vi "niFpga wdp fft DIT 16spc.vi"(0 "real data in":fxp<+/-,8,1>[](array[numeric])=[0.0, 0.0, 0.0, 0.0, 0.0, 0.0, 0.0, 0.0, 0.0, 0.0, 0.0, 0.0, 0.0, 0.0, 0.0, 0.0], 5 "imaginary data in":fxp<+/-,8,1>[](array[numeric])=[0.0, 0.0, 0.0, 0.0, 0.0, 0.0, 0.0, 0.0, 0.0, 0.0, 0.0, 0.0, 0.0, 0.0, 0.0, 0.0], 9 "input frame start":bool, 12 "enable":bool) -> (3 "data indices":u16[](array[numeric]), 4 "real data out":fxp<+,8,1>[](array[numeric]), 6 "imaginary data out":fxp<+,8,1>[](array[numeric]), 10 "output valid":bool, 14 "ready for frame":bool, 15 "output frame start":bool)   [LabVIEW 2017]
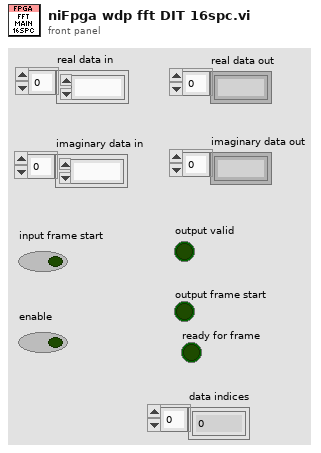
[diagram p1: front panel]
types:
  T1 = cluster{"internal input type":fxp<+/-,8,1>, "internal input type":fxp<+/-,8,1>}
  T2 = cluster{"twiddle factor type":fxp<+/-,16,2>, "twiddle factor type":fxp<+/-,16,2>}[]
  T3 = cluster{"x-y":fxp<+/-,19,12>, "x-y":fxp<+/-,19,12>}
  T4 = cluster{"x+y":fxp<+/-,19,12>, "x+y":fxp<+/-,19,12>}
  T5 = cluster{"x-y":fxp<+/-,19,12>, "x-y":fxp<+/-,19,12>}[]
  T6 = cluster{"x+y":fxp<+/-,19,12>, "x+y":fxp<+/-,19,12>}[]
  T7 = cluster{"data re":fxp<+/-,8,1>, "data im":fxp<+/-,8,1>}[]
  T8 = cluster{"x-y":fxp<+/-,20,13>, "x-y":fxp<+/-,20,13>}[]
  T9 = cluster{"x-y":fxp<+/-,20,13>, "x-y":fxp<+/-,20,13>}
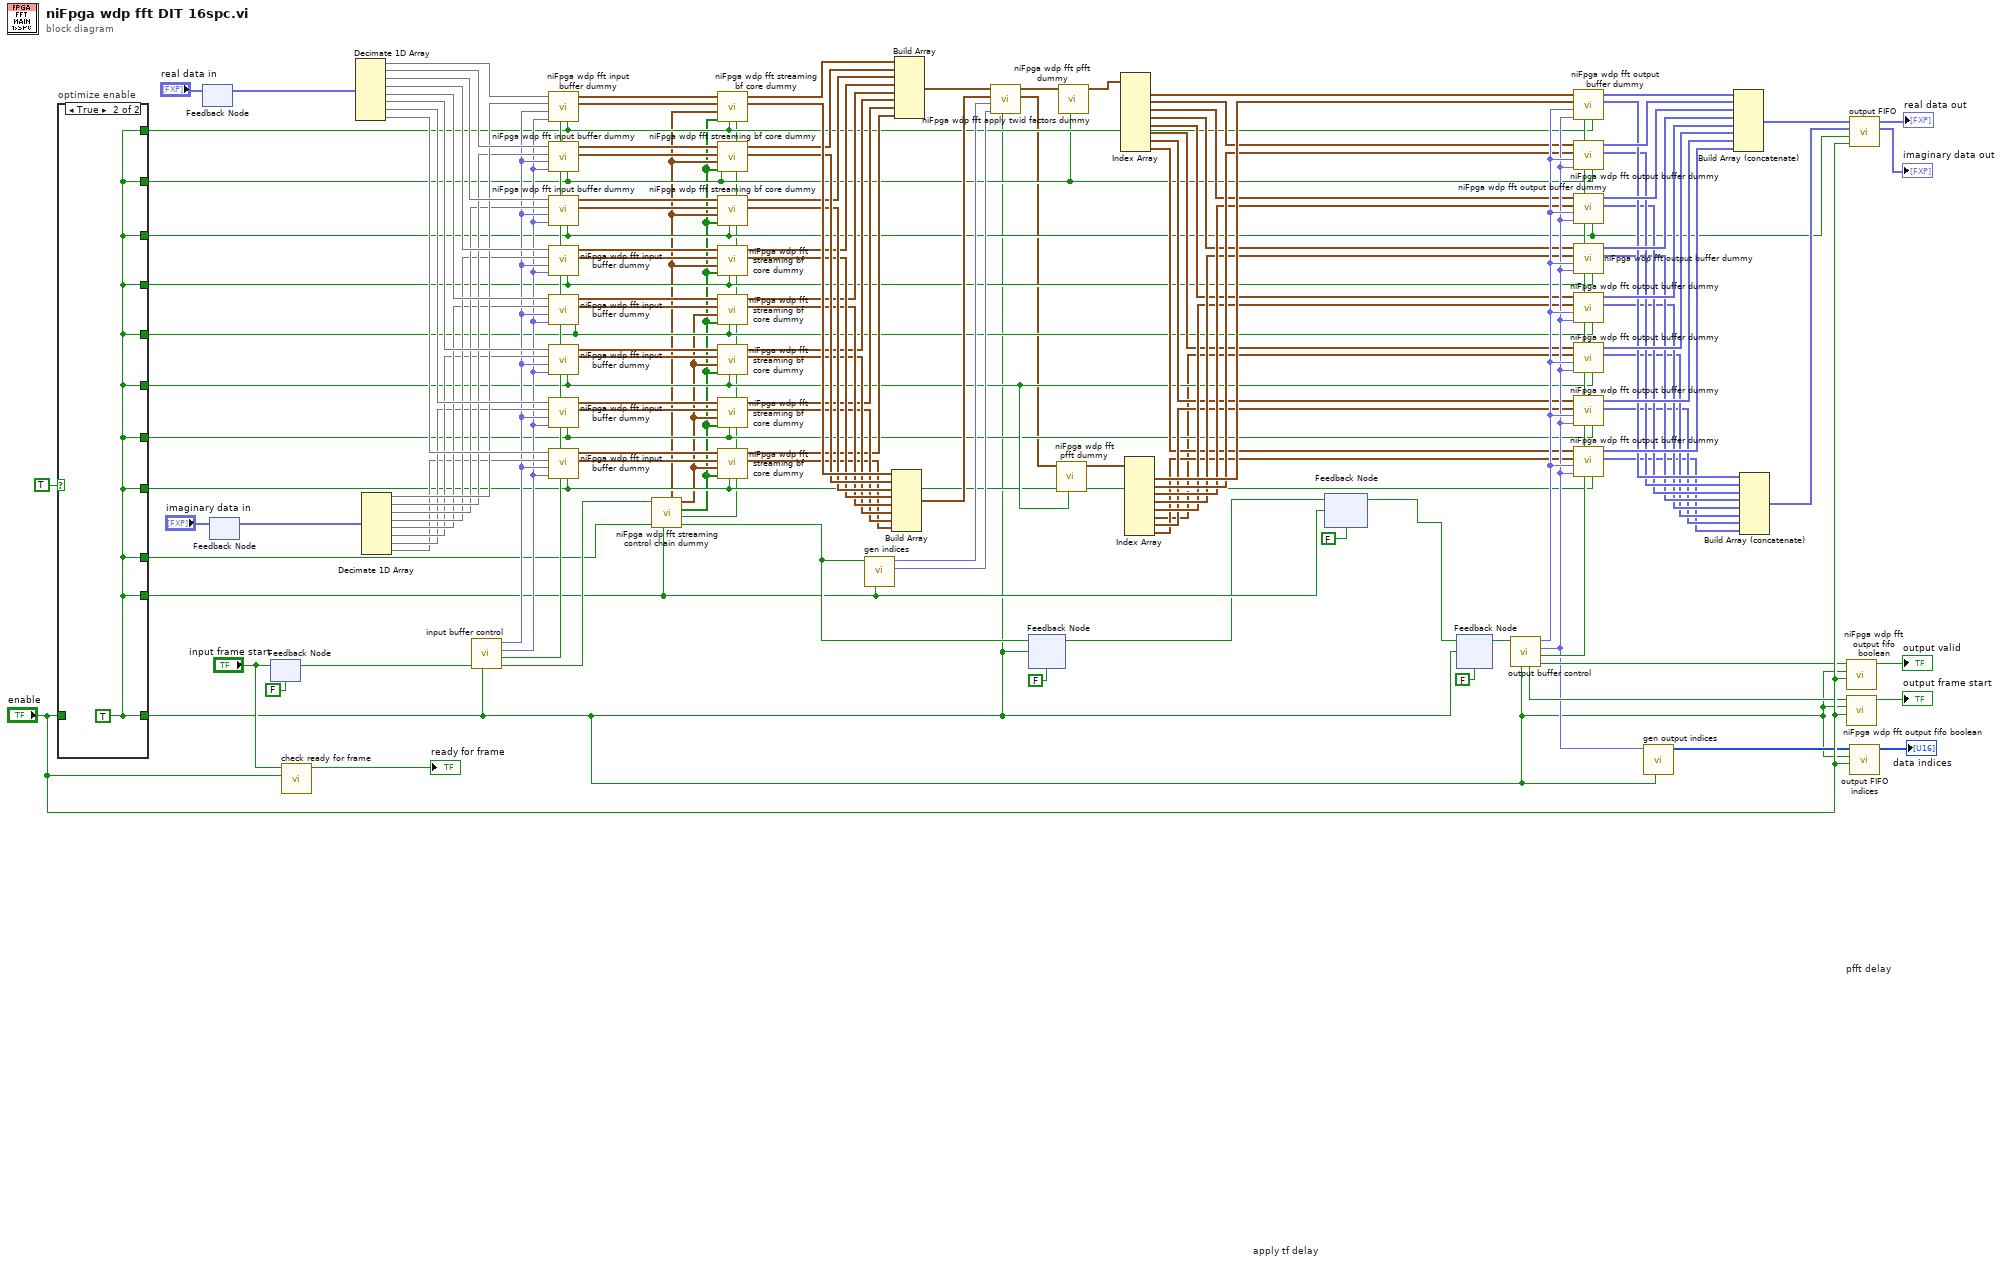
[diagram p0: block diagram]
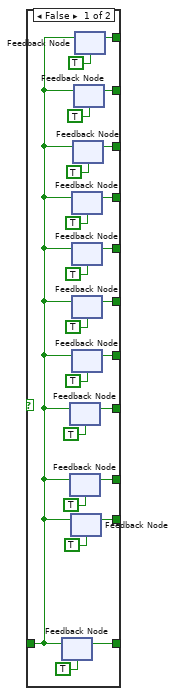
[diagram p2: hidden frame]
diagram:
  n1 = case "optimize enable" shown="True" TRUE {
    tunnel: [w159 w161] -> w9
    tunnel: [w157 w161] -> w13
    tunnel: [w148 w161] -> w24
    tunnel: [w147 w161] -> w23
    tunnel: [w146 w161] -> w22
    tunnel: [w145 w161] -> w21
    tunnel: [w144 w161] -> w20
    tunnel: [w143 w161] -> w19
    tunnel: [w142 w161] -> w18
    tunnel: [w141 w161] -> w17
    tunnel: "enable" -> [w139 _]
    tunnel: [w138 w161] -> w12
    frame False {
      n2 = feedback #1(TRUE ("enable")) -> (w159:bool)
      n3 = feedback-in #1(w139) -> ()
      n4 = feedback #2(TRUE ("enable")) -> (w141:bool)
      n5 = feedback-in #2(w139) -> ()
      n6 = feedback #3(TRUE ("enable")) -> (w138:bool)
      n7 = feedback-in #3(w139) -> ()
      n8 = feedback #4(TRUE ("enable")) -> (w157:bool)
      n9 = feedback-in #4(w139) -> ()
      n10 = feedback #5(TRUE ("enable")) -> (w145:bool)
      n11 = feedback-in #5(w139) -> ()
      n12 = feedback #6(TRUE ("enable")) -> (w144:bool)
      n13 = feedback-in #6(w139) -> ()
      n14 = feedback #7(TRUE ("enable")) -> (w143:bool)
      n15 = feedback-in #7(w139) -> ()
      n16 = feedback #8(TRUE ("enable")) -> (w142:bool)
      n17 = feedback-in #8(w139) -> ()
      n18 = feedback #9(TRUE ("enable")) -> (w146:bool)
      n19 = feedback-in #9(w139) -> ()
      n20 = feedback #10(TRUE ("enable")) -> (w147:bool)
      n21 = feedback-in #10(w139) -> ()
      n22 = feedback #11(TRUE ("enable")) -> (w148:bool)
      n23 = feedback-in #11(w139) -> ()
    }
    frame True {
      w161 = TRUE
    }
  }
  n24 = feedback #12() -> (w114:fxp<+/-,8,1>[])  [unwired: 1 in]
  n25 = feedback-in #12("real data in") -> ()
  n26 = feedback #13() -> (w105:fxp<+/-,8,1>[])  [unwired: 1 in]
  n27 = feedback-in #13("imaginary data in") -> ()
  n28 = feedback #14(FALSE ("enable")) -> (w132:bool)
  n29 = feedback-in #14("input frame start") -> ()
  n30 = call "check ready for frame"("enable"="enable", "frame start in"="input frame start") -> ("ready for frame"=→"ready for frame":bool)  [unwired: 9 in]
  n31 = Decimate 1D Array(w114) -> (w113:fxp<+/-,8,1>[], w112:fxp<+/-,8,1>[], w111:fxp<+/-,8,1>[], w110:fxp<+/-,8,1>[], w109:fxp<+/-,8,1>[], w108:fxp<+/-,8,1>[], w107:fxp<+/-,8,1>[], w106:fxp<+/-,8,1>[])
  n32 = Decimate 1D Array(w105) -> (w104:fxp<+/-,8,1>[], w103:fxp<+/-,8,1>[], w102:fxp<+/-,8,1>[], w101:fxp<+/-,8,1>[], w100:fxp<+/-,8,1>[], w99:fxp<+/-,8,1>[], w98:fxp<+/-,8,1>[], w97:fxp<+/-,8,1>[])
  n33 = call "input buffer control"("enable"=w9, "frame start in"=w132) -> ("frame start out"=w40:bool, "write memory 2?"=w89:bool, "read index"=w95:fxp<+,9,9>, "write index"=w96:fxp<+,8,8>)  [unwired: 6 in]
  n34 = call <vilib>:"niFpga wdp fft input buffer dummy.vi"("enable"=w24, "write memory 2?"=w89, "read index"=w95, "write index"=w96, "data in im"=w104, "data in re"=w113) -> ("data out 1"=w78:T1, "data out 0"=w79:T1)  [unwired: 4 in]
  n35 = call <vilib>:"niFpga wdp fft input buffer dummy.vi"("enable"=w23, "write memory 2?"=w89, "read index"=w95, "write index"=w96, "data in im"=w103, "data in re"=w112) -> ("data out 1"=w76:T1, "data out 0"=w77:T1)  [unwired: 4 in]
  n36 = call <vilib>:"niFpga wdp fft input buffer dummy.vi"("enable"=w22, "write memory 2?"=w89, "read index"=w95, "write index"=w96, "data in im"=w102, "data in re"=w111) -> ("data out 1"=w74:T1, "data out 0"=w75:T1)  [unwired: 4 in]
  n37 = call <vilib>:"niFpga wdp fft input buffer dummy.vi"("enable"=w21, "write memory 2?"=w89, "read index"=w95, "write index"=w96, "data in im"=w101, "data in re"=w110) -> ("data out 1"=w72:T1, "data out 0"=w73:T1)  [unwired: 4 in]
  n38 = call <vilib>:"niFpga wdp fft input buffer dummy.vi"("enable"=w20, "write memory 2?"=w89, "read index"=w95, "write index"=w96, "data in im"=w100, "data in re"=w109) -> ("data out 1"=w70:T1, "data out 0"=w71:T1)  [unwired: 4 in]
  n39 = call <vilib>:"niFpga wdp fft input buffer dummy.vi"("enable"=w19, "write memory 2?"=w89, "read index"=w95, "write index"=w96, "data in im"=w99, "data in re"=w108) -> ("data out 1"=w68:T1, "data out 0"=w69:T1)  [unwired: 4 in]
  n40 = call <vilib>:"niFpga wdp fft input buffer dummy.vi"("enable"=w18, "write memory 2?"=w89, "read index"=w95, "write index"=w96, "data in im"=w98, "data in re"=w107) -> ("data out 1"=w66:T1, "data out 0"=w67:T1)  [unwired: 4 in]
  n41 = call <vilib>:"niFpga wdp fft input buffer dummy.vi"("enable"=w17, "write memory 2?"=w89, "read index"=w95, "write index"=w96, "data in im"=w97, "data in re"=w106) -> ("data out 1"=w64:T1, "data out 0"=w65:T1)  [unwired: 4 in]
  n42 = call <vilib>:"niFpga wdp fft streaming control chain dummy.vi"("enable"=w13, "enable 1"=w12, "input frame start"=w40) -> ("frame start"=w14:bool, "index=0?"=w7:bool, "switch"=w4:bool[], "twiddle factors 1"=w5:T2, "twiddle factors"=w6:T2)  [unwired: 4 in]
  n43 = call <vilib>:"niFpga wdp fft streaming bf core dummy.vi"("index=0?"=w7, "enable"=w24, "switch"=w4, "twiddle factors"=w6, "data in 1"=w78, "data in 0"=w79) -> ("data out 1"=w59:T3, "data out 0"=w60:T4)  [unwired: 4 in]
  n44 = call <vilib>:"niFpga wdp fft streaming bf core dummy.vi"("index=0?"=w7, "enable"=w23, "switch"=w4, "twiddle factors"=w6, "data in 1"=w76, "data in 0"=w77) -> ("data out 1"=w57:T3, "data out 0"=w58:T4)  [unwired: 4 in]
  n45 = call <vilib>:"niFpga wdp fft streaming bf core dummy.vi"("index=0?"=w7, "enable"=w22, "switch"=w4, "twiddle factors"=w6, "data in 1"=w74, "data in 0"=w75) -> ("data out 1"=w55:T3, "data out 0"=w56:T4)  [unwired: 4 in]
  n46 = call <vilib>:"niFpga wdp fft streaming bf core dummy.vi"("index=0?"=w7, "enable"=w21, "switch"=w4, "twiddle factors"=w6, "data in 1"=w72, "data in 0"=w73) -> ("data out 1"=w53:T3, "data out 0"=w54:T4)  [unwired: 4 in]
  n47 = call <vilib>:"niFpga wdp fft streaming bf core dummy.vi"("index=0?"=w7, "enable"=w20, "switch"=w4, "twiddle factors"=w5, "data in 1"=w70, "data in 0"=w71) -> ("data out 1"=w51:T3, "data out 0"=w52:T4)  [unwired: 4 in]
  n48 = call <vilib>:"niFpga wdp fft streaming bf core dummy.vi"("index=0?"=w7, "enable"=w19, "switch"=w4, "twiddle factors"=w5, "data in 1"=w68, "data in 0"=w69) -> ("data out 1"=w49:T3, "data out 0"=w50:T4)  [unwired: 4 in]
  n49 = call <vilib>:"niFpga wdp fft streaming bf core dummy.vi"("index=0?"=w7, "enable"=w18, "switch"=w4, "twiddle factors"=w5, "data in 1"=w66, "data in 0"=w67) -> ("data out 1"=w47:T3, "data out 0"=w48:T4)  [unwired: 4 in]
  n50 = call <vilib>:"niFpga wdp fft streaming bf core dummy.vi"("index=0?"=w7, "enable"=w17, "switch"=w4, "twiddle factors"=w5, "data in 1"=w64, "data in 0"=w65) -> ("data out 1"=w45:T3, "data out 0"=w46:T4)  [unwired: 4 in]
  n51 = call "gen indices"("enable"=w13, "frame start"=w14) -> ("data index 1"=w41:fxp<+,10,10>, "data index 0"=w42:fxp<+,10,10>)  [unwired: 8 in]
  n52 = Build Array(w59, w57, w55, w53, w51, w49, w47, w45) -> (w44:T5)
  n53 = Build Array(w60, w58, w56, w54, w52, w50, w48, w46) -> (w63:T6)
  n54 = call <vilib>:"niFpga wdp fft apply twid factors dummy.vi"("enable"=w9, "data index 1"=w41, "data index 0"=w42, "data in 1"=w44, "data in 0"=w63) -> ("data out 1"=w2:T7, "data out 0"=w3:T7)  [unwired: 5 in]
  n55 = feedback #15 "apply tf delay"(FALSE) -> (w8:bool)
  n56 = feedback-in #15(w14, w9) -> ()
  n57 = call <vilib>:"niFpga wdp fft pfft dummy.vi"("enable"=w19, "data in"=w2) -> ("data out"=w61:T8)  [unwired: 9 in]
  n58 = call <vilib>:"niFpga wdp fft pfft dummy.vi"("enable"=w23, "data in"=w3) -> ("data out"=w62:T8)  [unwired: 9 in]
  n59 = Index Array(array=w62) -> (element #1=w39:T9, element #2=w37:T9, element #3=w35:T9, element #4=w33:T9, element #5=w31:T9, element #6=w29:T9, element #7=w28:T9, element #8=w26:T9)  [unwired: 8 in]
  n60 = Index Array(array=w61) -> (element #1=w38:T9, element #2=w36:T9, element #3=w34:T9, element #4=w32:T9, element #5=w30:T9, element #6=w16:T9, element #7=w27:T9, element #8=w25:T9)  [unwired: 8 in]
  n61 = feedback #16 "pfft delay"(FALSE) -> (w11:bool)
  n62 = feedback-in #16(w8, w13) -> ()
  n63 = feedback #17 ("delay")(FALSE) -> (w10:bool)
  n64 = feedback-in #17(w11, w9) -> ()
  n65 = call "output buffer control"("enable"=w9, "frame start"=w10) -> ("output valid?"=w85:bool, "memory switch"=w82:bool, "read index"=w81:fxp<+,4,4>, "write index"=w83:fxp<+,9,9>, "frame start?"=w84:bool)  [unwired: 5 in]
  n66 = call <vilib>:"niFpga wdp fft output buffer dummy.vi"("enable"=w24, "memory switch"=w82, "read index"=w81, "write index"=w83, "data in 1"=w38, "data in 0"=w39) -> ("data out im"=w122:fxp<+/-,32,16>[], "data out re"=w130:fxp<+/-,32,16>[])  [unwired: 4 in]
  n67 = call <vilib>:"niFpga wdp fft output buffer dummy.vi"("enable"=w23, "memory switch"=w82, "read index"=w81, "write index"=w83, "data in 1"=w36, "data in 0"=w37) -> ("data out im"=w121:fxp<+/-,32,16>[], "data out re"=w129:fxp<+/-,32,16>[])  [unwired: 4 in]
  n68 = call <vilib>:"niFpga wdp fft output buffer dummy.vi"("enable"=w22, "memory switch"=w82, "read index"=w81, "write index"=w83, "data in 1"=w34, "data in 0"=w35) -> ("data out im"=w120:fxp<+/-,32,16>[], "data out re"=w128:fxp<+/-,32,16>[])  [unwired: 4 in]
  n69 = call <vilib>:"niFpga wdp fft output buffer dummy.vi"("enable"=w21, "memory switch"=w82, "read index"=w81, "write index"=w83, "data in 1"=w32, "data in 0"=w33) -> ("data out im"=w119:fxp<+/-,32,16>[], "data out re"=w127:fxp<+/-,32,16>[])  [unwired: 4 in]
  n70 = call <vilib>:"niFpga wdp fft output buffer dummy.vi"("enable"=w20, "memory switch"=w82, "read index"=w81, "write index"=w83, "data in 1"=w30, "data in 0"=w31) -> ("data out im"=w118:fxp<+/-,32,16>[], "data out re"=w126:fxp<+/-,32,16>[])  [unwired: 4 in]
  n71 = call <vilib>:"niFpga wdp fft output buffer dummy.vi"("enable"=w19, "memory switch"=w82, "read index"=w81, "write index"=w83, "data in 1"=w16, "data in 0"=w29) -> ("data out im"=w117:fxp<+/-,32,16>[], "data out re"=w125:fxp<+/-,32,16>[])  [unwired: 4 in]
  n72 = call <vilib>:"niFpga wdp fft output buffer dummy.vi"("enable"=w18, "memory switch"=w82, "read index"=w81, "write index"=w83, "data in 1"=w27, "data in 0"=w28) -> ("data out im"=w116:fxp<+/-,32,16>[], "data out re"=w124:fxp<+/-,32,16>[])  [unwired: 4 in]
  n73 = call <vilib>:"niFpga wdp fft output buffer dummy.vi"("enable"=w17, "memory switch"=w82, "read index"=w81, "write index"=w83, "data in 1"=w25, "data in 0"=w26) -> ("data out im"=w115:fxp<+/-,32,16>[], "data out re"=w123:fxp<+/-,32,16>[])  [unwired: 4 in]
  n74 = call "gen output indices"("enable"=w9, "index"=w81) -> ("data indices"=w80:u16[])  [unwired: 9 in]
  n75 = Build Array (concatenate)(w130, w129, w128, w127, w126, w125, w124, w123) -> (w93:fxp<+/-,32,16>[])
  n76 = Build Array (concatenate)(w122, w121, w120, w119, w118, w117, w116, w115) -> (w91:fxp<+/-,32,16>[])
  n77 = call <vilib>:"niFpga wdp fft output fifo boolean.vi"("enable"="enable", "enable with delay"=w9, "boolean in"=w85) -> ("boolean out"=→"output valid":bool)  [unwired: 8 in]
  n78 = call <vilib>:"niFpga wdp fft output fifo boolean.vi"("enable"="enable", "enable with delay"=w9, "boolean in"=w84) -> ("boolean out"=→"output frame start":bool)  [unwired: 8 in]
  n79 = call "output FIFO"("enable"="enable", "enable with delay"=w22, "data in 1"=w91, "data in 0"=w93) -> ("data out 1"=→"imaginary data out":fxp<+,8,1>[], "data out 0"=→"real data out":fxp<+,8,1>[])  [unwired: 6 in]
  n80 = call "output FIFO indices"("enable"="enable", "enable with delay"=w9, "data in"=w80) -> ("data out"=→"data indices":u16[])  [unwired: 8 in]
